vi "VPPW Vapor Pressure of Pure Water (Pa).vi"(1 "Tceg":dbl[unit]) -> (0 "VPPW":dbl[unit])   [LabVIEW 2018]
panel:
  out "Temprature of Pure Water \nKelvin Degree":dbl[unit](slide) scale=273.0..373.0
  out "Tk":dbl[unit]
  out "Temprature of Pure Water\nCentigrade Degree":dbl[unit](slide) scale=0.0..100.0
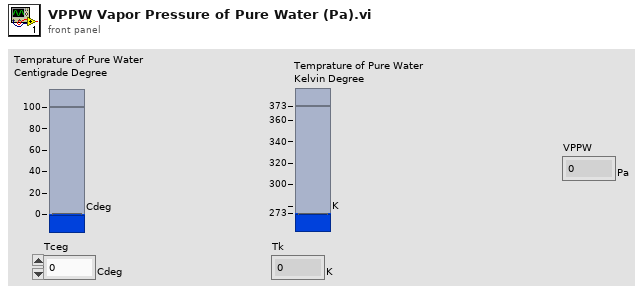
[diagram p1: front panel]
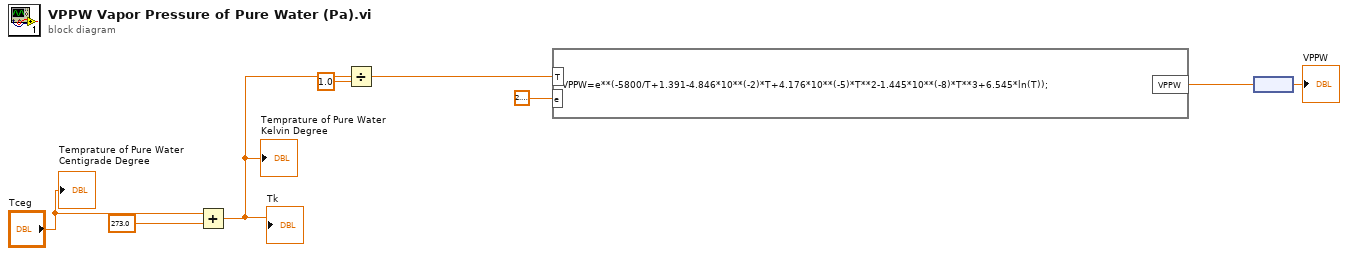
[diagram p0: block diagram]
diagram:
  n1 = Add(x="Tceg", y=dbl[unit] 273.0) -> (x+y=w3:dbl[unit])
  "Tk" <- w3
  "Temprature of Pure Water \nKelvin Degree" <- w3
  n2 = Divide(x=w3, y=dbl[unit] 1.0) -> (x/y=w8:dbl)
  n3 = formula code="VPPW=e**(-5800/T+1.391-4.846*10**(-2)*T+4.176*10**(-5)*T**2-1.445*10**(-8)*T**3+6.545*ln(T));"("T"=w8, "e"=2.718281828459045) -> ("VPPW"=w6:dbl)
  n4 = node(w6) -> (→"VPPW":dbl[unit])
  "Temprature of Pure Water\nCentigrade Degree" <- "Tceg"
